vi "Config-Sweep-Secondary Sour.vi"(5 "power compliance (0 = OFF)":dbl format="%^.2e", 6 "compliance":dbl=2.0 format="%^.2e", 7 "step":dbl=2e-05 format="%^.4e", 8 "error in (no error)":errorcluster, 9 "total points":i32=1, 10 "start":dbl=2e-05 format="%^.4e", 11 "VISA session":refnum<visa-resource-name>) -> (0 "error out":errorcluster, 3 "VISA resource name out":refnum<visa-resource-name>)   [LabVIEW 2016, in "Agilent 415X Series.lvlib"]
doc: "This VI configures the secondary sweep source (VAR2) for a sweep mode measurement. \n* This VI does not perform error checking on MEASUREMENT MODE or UNIT TYPE of VAR2, therefore it is the application programmer's responsibility to make certain this VI is used in the proper mode."
uses:
  Agilent 415X Series.lvlib
panel:
  # "This VI should be used only when a secondary\nsource (SMU or VSU) is specified."
  # "(W)"
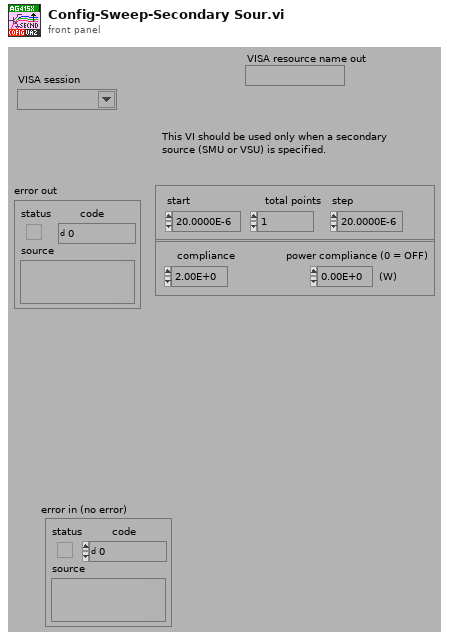
[diagram p1: front panel]
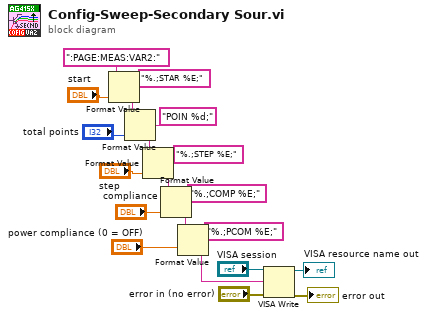
[diagram p0: block diagram]
diagram:
  n1 = Format Value(string ("")=":PAGE:MEAS:VAR2:", format string="%.;STAR %E;", value (0)="start") -> (output string=w17:string)
  n2 = Format Value(string ("")=w17, format string="POIN %d;", value (0)="total points") -> (output string=w6:string)
  n3 = Format Value(string ("")=w6, format string="%.;STEP %E;", value (0)="step") -> (output string=w3:string)
  n4 = Format Value(string ("")=w3, format string="%.;COMP %E;", value (0)="compliance") -> (output string=w2:string)
  n5 = Format Value(string ("")=w2, format string="%.;PCOM %E;", value (0)="power compliance (0 = OFF)") -> (output string=w12:string)
  n6 = VISA Write(VISA resource name="VISA session", write buffer=w12, error in (no error)="error in (no error)") -> (VISA resource name out=→"VISA resource name out":refnum<visa-resource-name>, error out=→"error out":errorcluster)  [unwired: 1 out]
